vi "Get Screen Size v1.vi"(8 "error in (no error)":errorcluster) -> (0 "error out":errorcluster, 2 "Width":i32, 3 "Height":i32)   [LabVIEW 2014]
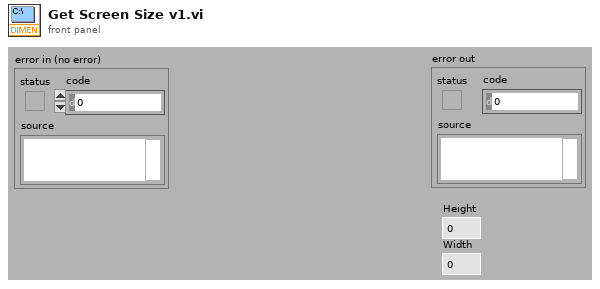
[diagram p1: front panel]
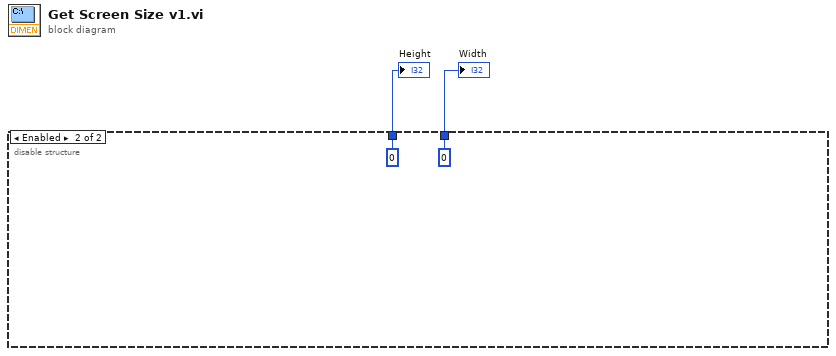
[diagram p0: block diagram]
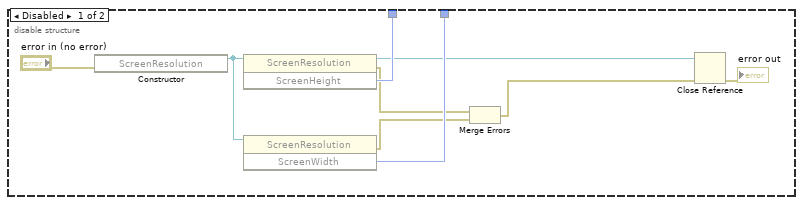
[diagram p2: hidden frame]
diagram:
  n1 = disable-structure shown="Enabled" {
    disable-tunnel: [w9 0 ("Height")] -> w2
    disable-tunnel: [w8 0 ("Width")] -> w1
    frame Disabled {
      n2 = constructor class="ScreenResolution"(error in="error in (no error)") -> (reference out=w11:refnum<k24>)  [unwired: 2 in, 2 out]
      n3 = invoke class="ScreenResolution" method="ScreenHeight"(reference=w11) -> (reference out=w4:refnum<k24>, error out=w5:errorcluster, "ScreenHeight"=w9:i32)  [unwired: 2 in]
      n4 = invoke class="ScreenResolution" method="ScreenWidth"(reference=w11) -> (error out=w7:errorcluster, "ScreenWidth"=w8:i32)  [unwired: 2 in, 1 out]
      n5 = Merge Errors(w5, w7) -> (w6:errorcluster)
      n6 = Close Reference(reference=w4, error in (no error)=w6) -> (error out=→"error out":errorcluster)
    }
    frame Enabled {
    }
  }
  "Height" <- w2
  "Width" <- w1
